vi "auto datalogger.vi"(9 "data log interval (s)":u32=1 min=1, 11 "Datalog directory path":path) -> (0 "File Failure":bool, 3 "File refnum":refnum<file>)   [LabVIEW 2015]
uses:
  DAQ configuration/Sensor buffer command.ctl
  logic buffer cmd.ctl
  calibration/Shared Data/buffer.ctl
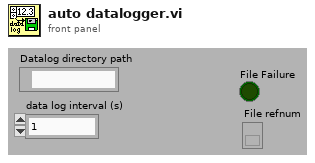
[diagram p1: front panel]
types:
  T1 = typedef "buffer.ctl" = enum16{"write", "read", "read merge"}
  T2 = typedef "logic buffer cmd.ctl" = enum16{"read", "write ouput settings", "write rules", "write setpoints", "write output descriptions", "write all", "calculate setpoints", "save", "open", "Load all setpoint code", "Load one setpoint code", "Configure one setpoint code"}
  T3 = typedef "Sensor buffer command.ctl" = enum16{"read average", "read recent", "read all", "write", "set buffer size", "Read channel config", "Write channel config", "clear"}
  T4 = enum16{"open", "open or create", "create or replace", "create", "open (read only)"}
  T5 = typedef "variable setpoint.ctl" = cluster{"name":string, "unit":string, "value":dbl, "Type":enum16{"Constant", "Variable"}, "variable":cluster{"selected sensors":i32[], "selected set points":i32[], "VI":path, "Data average interval":T6, "code ref":T7}}
  T6 = typedef "data ave interval.ctl" = dbl
  T7 = typedef "type specifier for control code.ctl" = refnum<vi>
  T8 = typedef "Sensor data.ctl" = cluster{" Sensor array":T9[], "Time":dbl}
  T9 = typedef "sensor cluster.ctl" = cluster{"voltage":sgl, "scaled":sgl, "units":string, "Out of Range":bool}
  T10 = typedef "Channel config.ctl" = cluster{"Channel Indices":T11[], "AI Max voltage":dbl[], "Calibration matrix":T12}
  T11 = typedef "channel identifier.ctl" = u16
  T12 = typedef "calib array.ctl" = T13[]
  T13 = typedef "conversion.ctl" = cluster{"conversion matrix":sgl[][], "units":string, "name":string, "scale type":T14, "offset (volts)":dbl, "second channel":i8, "correspondence table":T15, "offset (physical units)":dbl, "pH scale":T16, "D.O.":T17, "Photometer data":T18}
  T14 = typedef "scale type.ctl" = enum16{"Volts", "Polynomial", "Correspondence Table", "pH", "Dissolved Oxygen", "Quadratic", "Photometer"}
  T15 = typedef "correspondence table.ctl" = cluster{"physical units":dbl, "volts":dbl}[]
  T16 = typedef "pH scale.ctl" = cluster{"Buffers":cluster{"Buffer":dbl, "Calibrated":bool, "V/T":dbl}[], "Temperature":dbl}
  T17 = typedef "DO scale.ctl" = cluster{"Temperature":dbl, "K":dbl, "barometric pressure":dbl}
  T18 = typedef "Photometer calibration data.ctl" = cluster{"Dark Voltage":dbl, "Blank Voltage":dbl, "Standards":cluster{"Concentration":dbl, "Voltage":dbl}[]}
  T19 = cluster{string[], "Calibration matrix":T12, "Shared data names (unit) out":string[]}
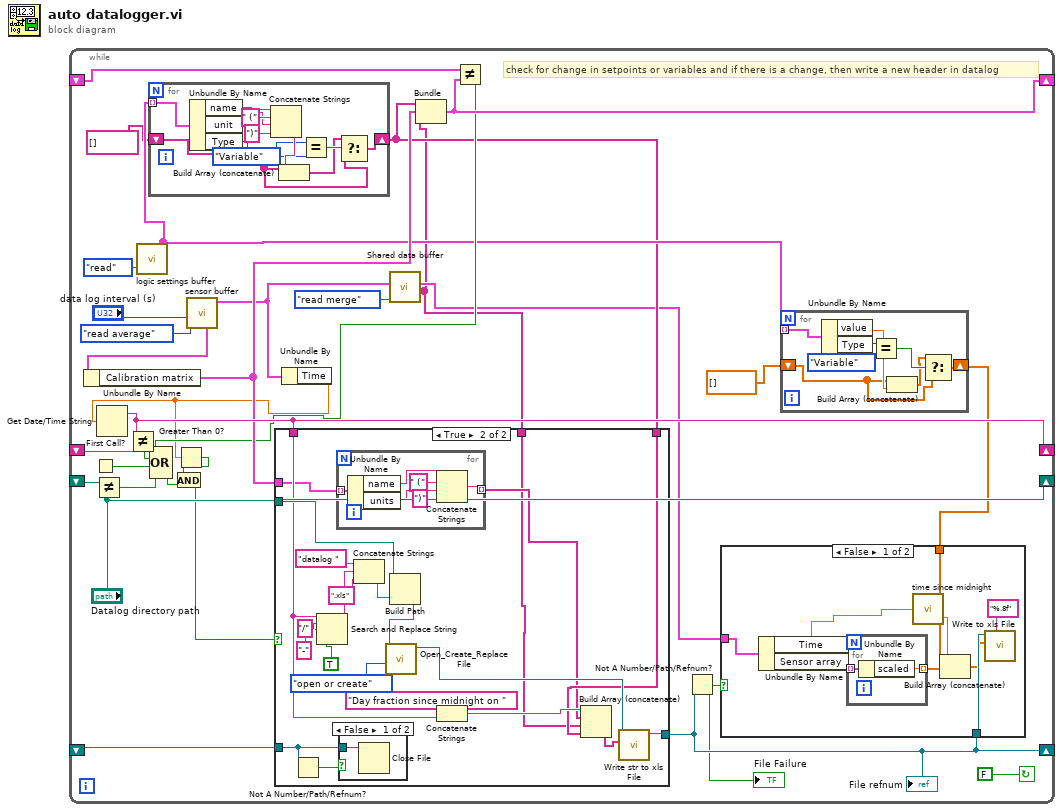
[diagram p0: block diagram]
diagram:
  n1 = while {
    shift-left: _ -> [w32]
    shift-right: ["Datalog directory path"] -> _
    shift-right: [w23] -> _
    shift-left: _ -> [w30]
    shift-right: [w25] -> _
    shift-left: _ -> [w24]
    shift-right: [w13] -> _
    shift-left: _ -> [w14]
    stop <- FALSE continue-if-true
    # "check for change in setpoints or variables and if there is a change, then write a new header in datalog"
    n2 = First Call?() -> (First Call?: T/F=w28:bool)
    n3 = Not Equal?(x=w32, y="Datalog directory path") -> (x != y?=w27:bool)
    n4 = call "logic settings buffer.vi"("command"=logic_buffer_cmd."read") -> ("Set Points out"=w11:T5[])  [unwired: 11 in, 7 out]
    n5 = for {
      tunnel: w11 -> [w44] mode=indexing
      shift-right: [w33] -> w9
      shift-left: string[] [] -> [w34]
      n6 = Unbundle By Name(w44) -> ("name"=w41:string, "unit"=w40:string, "Type"=w37:enum16{"Constant", "Variable"})
      n7 = Concatenate Strings(w41, " (" ("Substring"), w40, ")" ("Substring")) -> (w38:string)
      n8 = Build Array (concatenate)(w34, w38) -> (w35:string[])
      n9 = Equal?(x=w37, y=enum16{"Constant", "Variable"}."Variable") -> (x = y?=w39:bool)
      n10 = Select(t=w35, s=w39, f=w34) -> (s? t:f=w33:string[])
    }
    n11 = call "sensor buffer.vi"("command"=Sensor_buffer_command."read average", "smooth interval (s)"="data log interval (s)") -> ("Calibrated data"=w3:T8, "Channel Config out"=w16:T10)  [unwired: 5 in, 3 out]
    n12 = Unbundle By Name(w16) -> ("Calibration matrix"=w15:T12)
    n13 = Unbundle By Name(w3) -> ("Time"=w6:dbl)
    n14 = Get Date/Time String(seconds (now)=w6) -> (date string=w23:string)  [unwired: 2 in, 1 out]
    n15 = Not Equal?(x=w23, y=w30) -> (x != y?=w29:bool)
    n16 = Greater Than 0?(x=w6) -> (x > 0?=w5:bool)
    n17 = call "Shared data buffer.vi"("command"=buffer."read merge", "Data from local sources in"=w3) -> ("Shared data names (unit) out"=w1:string[], "Data from merged sources out"=w2:T8)  [unwired: 7 in, 1 out]
    n18 = Bundle(w9, "Calibration matrix"=w15, "Shared data names (unit) out"=w1) -> (w13:T19)  [unwired: 1 in]
    n19 = Not Equal?(x=w14, y=w13) -> (x != y?=w12:bool)
    n20 = Compound Arithmetic op=OR(w12, w29, w28, w27) -> (w8:bool)
    n21 = And(x=w5, y=w8) -> (x .and. y?=w7:bool)
    n22 = case shown="True" w7 {
      tunnel: w24 -> [w53 w61]
      tunnel: [w53 w75] -> w25
      tunnel: "Datalog directory path" -> [_ w72]
      tunnel: w23 -> [_ w62]
      tunnel: w15 -> [_ w57]
      tunnel: w9 -> [_ w56]
      tunnel: w1 -> [_ w54]
      frame False {
      }
      frame True {
        n23 = Not A Number/Path/Refnum?(number/path/refnum=w61) -> (NaN/Path/Refnum?=w60:bool)
        n24 = Search and Replace String(replace all?=TRUE ("replace all? (F)"), input string=w62, search string="/", replace string="-" ("replace string (\"\")")) -> (result string=w69:string)  [unwired: 4 in, 3 out]
        n25 = for {
          tunnel: w57 -> [w82] mode=indexing
          tunnel: [w77] -> w55 mode=indexing
          n26 = Unbundle By Name(w82) -> ("name"=w81:string, "units"=w79:string)
          n27 = Concatenate Strings(w81, " (" ("Substring"), w79, ")" ("Substring")) -> (w77:string)
        }
        n28 = case shown="False" w60 {
          tunnel: w61 -> [w76 _]
          frame False {
            n29 = Close File(refnum=w76) -> ()  [unwired: 1 in, 2 out]
          }
          frame True {
          }
        }
        n30 = Concatenate Strings("datalog " ("string"), w69, ".xls" ("string")) -> (w68:string)
        n31 = Build Path(base path=w72, name or relative path=w68) -> (appended path=w67:path)
        n32 = call <vilib>:"Open_Create_Replace File.vi"("function (open:0)"=T4."open or create", "file path"=w67) -> ("refnum"=w65:refnum<file>)  [unwired: 6 in, 3 out]
        n33 = Concatenate Strings("Day fraction since midnight on " ("Substring"), w62) -> (w64:string)
        n34 = Build Array (concatenate)(w64, w55, w54, w56) -> (w59:string[])
        n35 = call "Write str to xls File.vi"("1D data"=w59, "refnum"=w65) -> ("dup refnum"=w75:refnum<file>)  [unwired: 8 in, 1 out]
      }
    }
    "File refnum" <- w25
    n36 = Not A Number/Path/Refnum?(number/path/refnum=w25) -> (NaN/Path/Refnum?=w22:bool)
    "File Failure" <- w22
    n37 = for {
      tunnel: w11 -> [w52] mode=indexing
      shift-right: [w46] -> w17
      shift-left: dbl[] [] -> [w45]
      n38 = Unbundle By Name(w52) -> ("value"=w48:dbl, "Type"=w51:enum16{"Constant", "Variable"})
      n39 = Equal?(x=w51, y=enum16{"Constant", "Variable"}."Variable") -> (x = y?=w49:bool)
      n40 = Build Array (concatenate)(w45, w48) -> (w47:dbl[])
      n41 = Select(t=w47, s=w49, f=w45) -> (s? t:f=w46:dbl[])
    }
    n42 = case shown="False" w22 {
      tunnel: w25 -> [w88 _]
      tunnel: w2 -> [w85 _]
      tunnel: w17 -> [w84 _]
      frame False {
        n43 = Unbundle By Name(w85) -> ("Time"=w87:dbl, "Sensor array"=w90:T9[])
        n44 = for {
          tunnel: w90 -> [w93] mode=indexing
          tunnel: [w92] -> w89 mode=indexing
          n45 = Unbundle By Name(w93) -> ("scaled"=w92:sgl)
        }
        n46 = call "time since midnight.vi"("seconds since 1Jan1904"=w87) -> ("Days"=w86:dbl)  [unwired: 1 out]
        n47 = Build Array (concatenate)(w86, w89, w84) -> (w83:dbl[])
        n48 = call "Write to xls File.vi"("format (%.3f)"="%.8f", "1D data"=w83, "refnum"=w88) -> ()  [unwired: 7 in, 2 out]
      }
      frame True {
      }
    }
  }
